vi "LC_BESS_global.vi"() -> ()   [LabVIEW 2016]
panel:
  in  "Digital control channel number":dbl
  in  "Digital statues channel number":dbl
  in  "Analogue control channel number":dbl
  in  "Analogue statues channel number":dbl
  in  "DNP3 Outstation Address":dbl
  in  "DNP3 Master Address":dbl
  in  "DNP3 port":dbl
  in  "IP_BESS":dbl[](array[numeric])
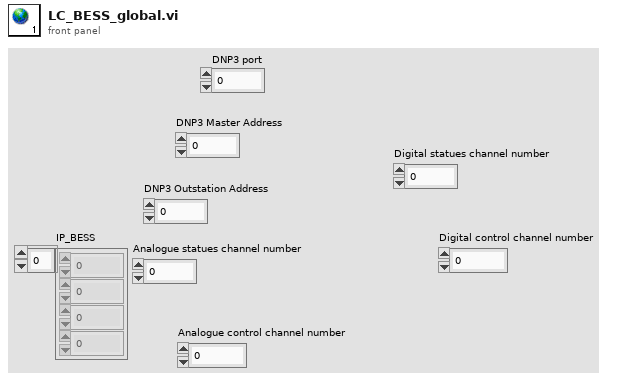
[diagram p1: front panel]
diagram:
